vi "FPGA Addon SysDef Example.vi"() -> ()   [LabVIEW 2019]
uses:
  NationalInstruments.VeriStand.Internal
  NationalInstruments.VeriStand.SystemDefinitionAPI
  FPGA System Definition API.lvlib
panel:
  out "Sysdef Path":path=path "C:/Users/Public/Documents/National Instruments/NI VeriStand 2015/Projects/DynamicallyCreatedProject/DynamicallyCreatedProject.nivssdf"
  in  "error in (no error)":errorcluster
  out "error out":errorcluster
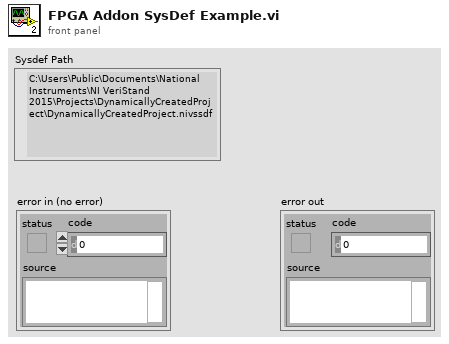
[diagram p1: front panel]
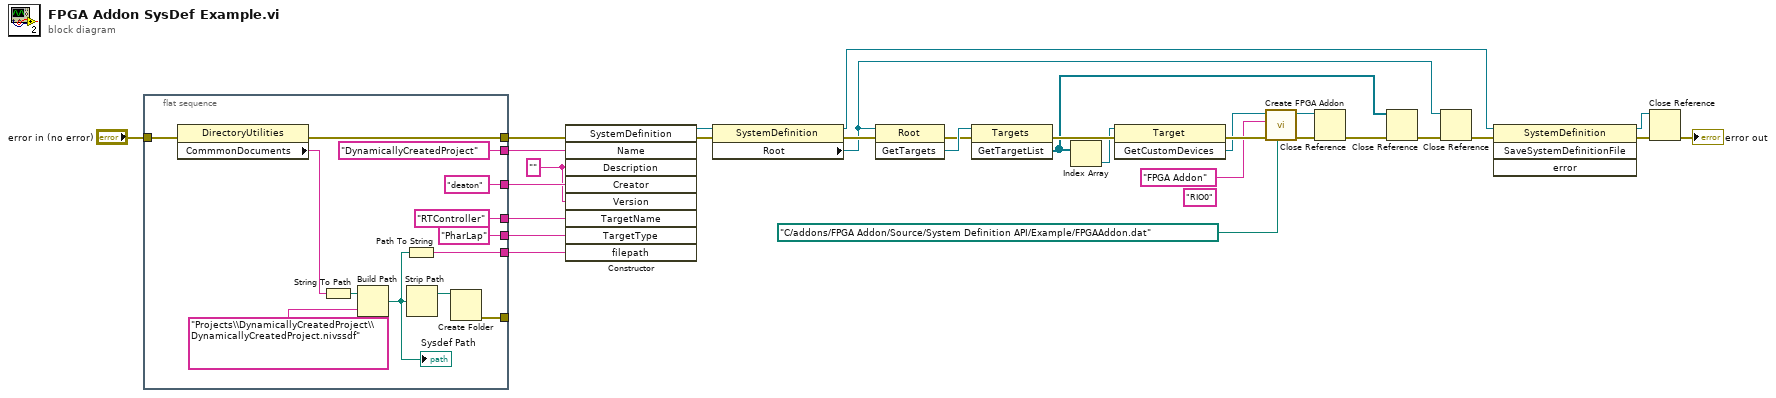
[diagram p0: block diagram]
diagram:
  (unwired) "RIO0" ("RIO Device")
  w27 = "" ("Description")
  n1 = flat-sequence {
    tunnel: ["DynamicallyCreatedProject" ("Name")] -> w30
    tunnel: ["deaton" ("Creator")] -> w29
    tunnel: ["PharLap" ("TargetType")] -> w28
    tunnel: [w40] -> w26
    tunnel: ["RTController" ("TargetName")] -> w20
    tunnel: "error in (no error)" -> [w33]
    tunnel: [w32] -> w6
    tunnel: [w31] -> _
    frame #0 {
      n2 = property class="DirectoryUtilities"(error in=w33) -> (error out=w32:errorcluster, "CommmonDocuments"=w37:string)  [unwired: 1 in, 1 out]
      n3 = String To Path(string=w37) -> (path=w36:path)
      n4 = Build Path(base path=w36, name or relative path="Projects\\DynamicallyCreatedProject\\DynamicallyCreatedProject.nivssdf") -> (appended path=w34:path)
      "Sysdef Path" <- w34
      n5 = Path To String(path=w34) -> (string=w40:string)
      n6 = Strip Path(path=w34) -> (stripped path=w38:path)  [unwired: 1 out]
      n7 = Create Folder(path (use dialog)=w38) -> (error out=w31:errorcluster)  [unwired: 2 in, 2 out]
    }
  }
  n8 = constructor class="SystemDefinition"(error in=w6, "Name"=w30, "Description"=w27, "Creator"=w29, "Version"=w27, "TargetName"=w20, "TargetType"=w28, "filepath"=w26) -> (reference out=w22:refnum<k24>, error out=w24:errorcluster)  [unwired: 2 in, 8 out]
  n9 = property class="SystemDefinition"(reference=w22, error in=w24) -> (reference out=w10:refnum<k24>, error out=w23:errorcluster, "Root"=w9:refnum<k24>)
  n10 = invoke class="Root" method="GetTargets"(reference=w9, error in=w23) -> (error out=w21:errorcluster, "GetTargets"=w25:refnum<k24>)  [unwired: 1 in, 1 out]
  n11 = invoke class="Targets" method="GetTargetList"(reference=w25, error in=w21) -> (error out=w19:errorcluster, "GetTargetList"=w8:refnum<k24>[])  [unwired: 1 in, 1 out]
  n12 = Index Array(array=w8) -> (element=w18:refnum<k24>)  [unwired: 1 in]
  n13 = invoke class="Target" method="GetCustomDevices"(reference=w18, error in=w19) -> (error out=w12:errorcluster, "GetCustomDevices"=w3:refnum<k24>)  [unwired: 1 in, 1 out]
  n14 = call "Create FPGA Addon.vi"("Configuration (.dat)"=path "C:/addons/FPGA Addon/Source/System Definition API/Example/FPGAAddon.dat" ("Path (.dat)"), "error in (no error)"=w12, "Name"="FPGA Addon", "Custom Devices Ref"=w3) -> ("error out"=w5:errorcluster, "Custom Devices Ref"=w11:refnum<k24>)  [unwired: 6 in]
  n15 = Close Reference(reference=w11, error in (no error)=w5) -> (error out=w4:errorcluster)
  n16 = Close Reference(reference=w8, error in (no error)=w4) -> (error out=w16:errorcluster)
  n17 = Close Reference(reference=w9, error in (no error)=w16) -> (error out=w17:errorcluster)
  n18 = invoke class="SystemDefinition" method="SaveSystemDefinitionFile"(reference=w10, error in=w17) -> (reference out=w15:refnum<k24>, error out=w13:errorcluster)  [unwired: 2 in, 2 out]
  n19 = Close Reference(reference=w15, error in (no error)=w13) -> (error out=→"error out":errorcluster)
